vi "WMS.vi"(0 "System no.":i32=1 min=1 max=4 step=1, 2 "Axes to set":string[](array[string]), 3 "Wave storage max.":i32[](array[numeric]), 5 "error in":errorcluster, 6 "Without axis ID?":bool) -> (14 "Controller error":bool, 19 "error out":errorcluster)   [LabVIEW 2020]
doc: "Sets maximum size of wave-point storage available for given axes and checks for error. If Without axis ID? is TRUE, then Axes to set is ignored and first field of Wave storage max. array is used as number of wave points for every axis. Controller error is TRUE if selected system reports error code which is not 0.\n\nE-710: Without axis ID? = FALSE. A maximum number of 63488 samples can be defined for all axes in total."
panel:
  # "Sets maximum size of wave-point storage available for given \naxes and checks for error. If Without axis ID? is TRUE, then Axes \nto set is ignored and first field of Wave storage max. array is used \nas number of wave points for every axis."
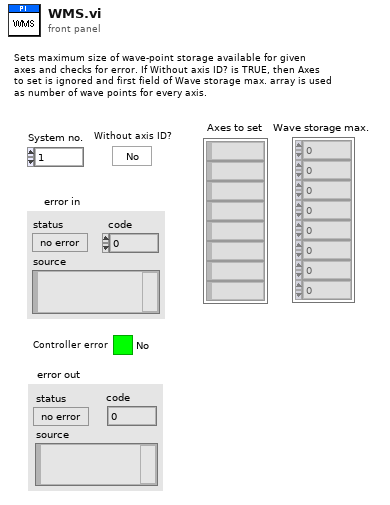
[diagram p1: front panel]
types:
  T1 = enum16{"Disable error check", "Force error check", "Use global settings"}
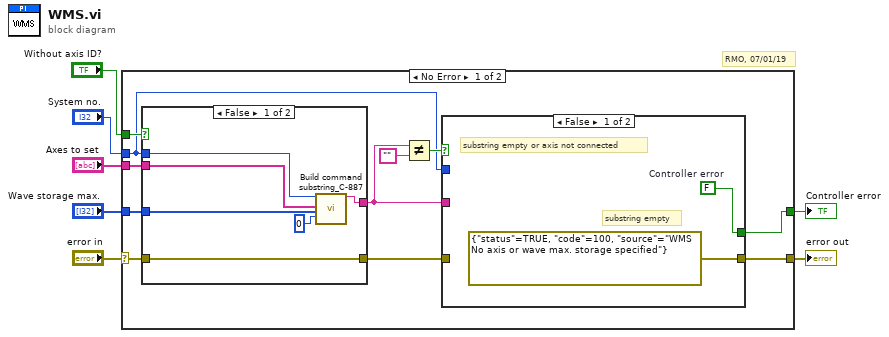
[diagram p0: block diagram]
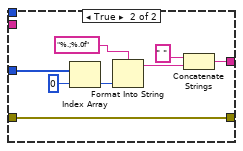
[diagram p2: hidden frame]
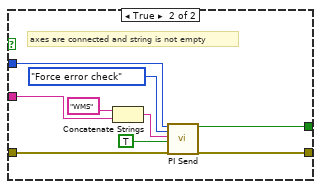
[diagram p3: hidden frame]
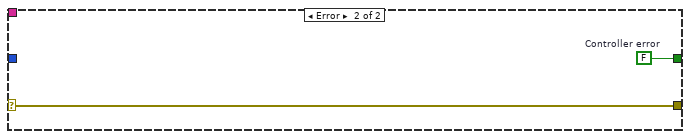
[diagram p4: hidden frame]
diagram:
  # "RMO, 07/01/19"
  n1 = case shown="No Error" "error in" {
    selector: "error in" -> [w9 w45]
    tunnel: [w18 w45] -> w7
    tunnel: "Wave storage max." -> [w15 _]
    tunnel: "System no." -> [w10 _]
    tunnel: "Axes to set" -> [w13 _]
    tunnel: "Without axis ID?" -> [w12 _]
    tunnel: [w8 w44] -> w1
    frame No Error {
      n2 = case shown="False" w12 {
        tunnel: [w24 w26] -> w16
        tunnel: w15 -> [w23 w25]
        tunnel: w9 -> [w20 w28]
        tunnel: [w20 w28] -> w14
        tunnel: w13 -> [w22 _]
        tunnel: w10 -> [w19 _]
        frame False {
          n3 = call "Build command substring_C-887.vi"("System no."=w19, "Affected axes"=w22, "Parameters"=w23, "No. of digits"=i16 0) -> ("Command substring"=w24:string)  [unwired: 3 in, 12 out]
        }
        frame True {
          n4 = Index Array(array=w25, index=0 ("Index")) -> (element=w31:i32)
          n5 = Format Into String(format string="%.;%.0f" ("Format String"), w31) -> (resulting string=w30:string)  [unwired: 2 in, 1 out]
          n6 = Concatenate Strings(" ", w30) -> (w26:string)
        }
      }
      n7 = Not Equal?(x=w16, y="") -> (x != y?=w11:bool)
      n8 = case shown="False" w11 {
        tunnel: w16 -> [_ w42]
        tunnel: [errorcluster {"status"=TRUE, "code"=100, "source"="WMS No axis or wave max. storage specified"} ("error out") w36] -> w18
        tunnel: w14 -> [_ w39]
        tunnel: w10 -> [_ w38]
        tunnel: [w33 w35] -> w8
        frame False {
          w33 = FALSE  # Controller error
          # "substring empty"
          # "substring empty or axis not connected"
        }
        frame True {
          # "axes are connected and string is not empty"
          n9 = Concatenate Strings("WMS", w42) -> (w40:string)
          n10 = call "PI Send.vi"("System no."=w38, "Error check settings"=T1."Force error check", "String to send"=w40, "Attach termination char.?"=TRUE ("Attach Linefeed?"), "error in"=w39) -> ("Controller error"=w35:bool, "error out"=w36:errorcluster)  [unwired: 1 in, 12 out]
        }
      }
    }
    frame Error {
      w44 = FALSE  # Controller error
    }
  }
  "error out" <- w7
  "Controller error" <- w1
